vi "plotToString.vi"(4 "Error Bar upper":string[](array[string]), 5 "Error Bar Type":T1, 6 "Error Bar lower":string[](array[string]), 7 "Transpose":bool, 8 "Precision2":string, 9 "Precision1":string, 10 "Column2":dbl[](array[numeric]), 11 "Column1":dbl[](array[numeric])) -> (2 "nLoops":i32, 3 "plotString":string)   [LabVIEW 2016]
uses:
  Error bar Type.ctl
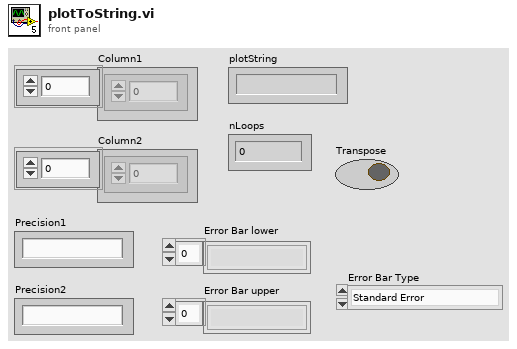
[diagram p1: front panel]
types:
  T1 = typedef "Error bar Type.ctl" = enum16{"Standard Error", "Separate upper and lower"}
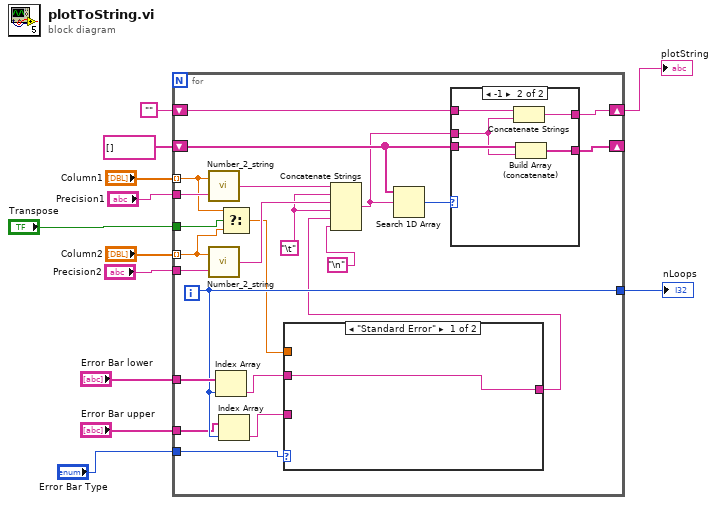
[diagram p0: block diagram]
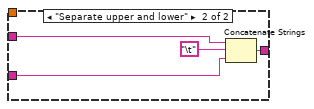
[diagram p2: hidden frame]
diagram:
  n1 = for {
    tunnel: "Column1" -> [w19] mode=indexing
    shift-right: [w32] -> w5
    shift-left: "" -> [w33]
    tunnel: "Column2" -> [w18] mode=indexing
    shift-right: [w31] -> _
    shift-left: string[] [] -> [w30]
    tunnel: "Precision1" -> [w27]
    tunnel: "Precision2" -> [w26]
    tunnel: [w24] -> w12
    tunnel: "Error Bar lower" -> [w25]
    tunnel: "Error Bar upper" -> [w23]
    tunnel: "Transpose" -> [w20]
    tunnel: "Error Bar Type" -> [w13]
    i -> [w24]
    w22 = "\t"
    n2 = call "Number_2_string.vi"("precision"=w27, "number"=w19) -> ("String"=w35:string)
    n3 = call "Number_2_string.vi"("precision"=w26, "number"=w18) -> ("String"=w34:string)
    n4 = Index Array(array=w25, index=w24) -> (element=w16:string)
    n5 = Index Array(array=w23, index=w24) -> (element=w15:string)
    n6 = Select(t=w19, s=w20, f=w18) -> (s? t:f=w17:dbl)
    n7 = case shown="\"Standard Error\"" w13 {
      tunnel: w17 -> [_ _]
      tunnel: w16 -> [w36 w38]
      tunnel: w15 -> [_ w37]
      tunnel: [w36 w39] -> w14
      frame "Standard Error" {
      }
      frame "Separate upper and lower" {
        n8 = Concatenate Strings(w38, "\t", w37) -> (w39:string)
      }
    }
    n9 = Concatenate Strings(w35, w22, w34, w22, w14, "\n") -> (w29:string)
    n10 = Search 1D Array(1D array=w30, element=w29) -> (index of element=w28:i32)  [unwired: 1 in]
    n11 = case shown="-1" w28 {
      tunnel: w33 -> [w42 w47]
      tunnel: [w42 w46] -> w32
      tunnel: w29 -> [_ w43]
      tunnel: w30 -> [w41 w45]
      tunnel: [w41 w44] -> w31
      frame 0, Default {
      }
      frame -1 {
        n12 = Concatenate Strings(w47, w43) -> (w46:string)
        n13 = Build Array (concatenate)(w45, w43) -> (w44:string[])
      }
    }
  }
  "nLoops" <- w12
  "plotString" <- w5
